vi "ResetAlarms.vi"(0 "reference in":refnum<class "Stand.lvclass">, 11 "error in (no error)":errorcluster) -> (4 "reference out":refnum<class "Stand.lvclass">, 15 "error out":errorcluster)   [LabVIEW 2019, in "Stand.lvclass"]
uses:
  Stand.lvclass
  Stand.lvclass/Stand.ctl
  Sig_AI_class/Sig_AI.lvclass
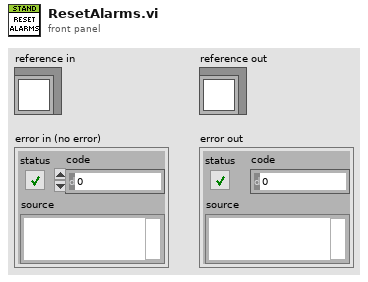
[diagram p1: front panel]
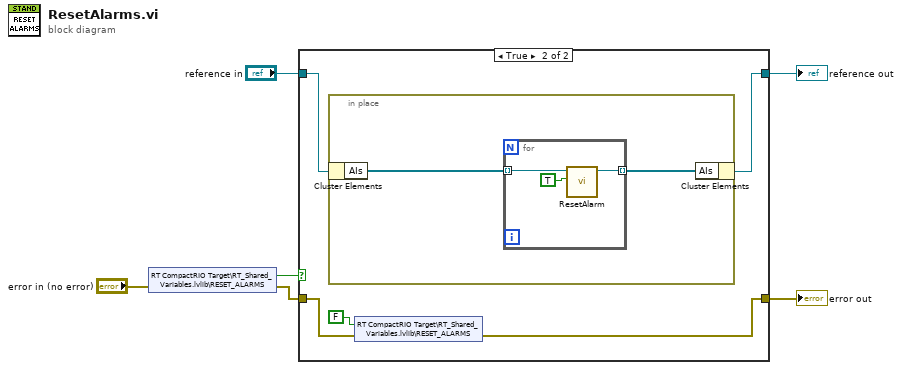
[diagram p0: block diagram]
diagram:
  n1 = shared-variable "RT CompactRIO Target\\RT_Shared_Variables.lvlib\\RESET_ALARMS"(error in="error in (no error)") -> (w2:bool, error out=w3:errorcluster)
  n2 = case shown="True" w2 {
    tunnel: w3 -> [w7 w12]
    tunnel: [w7 w11] -> w4
    tunnel: [w8 w9] -> w5
    tunnel: "reference in" -> [w8 w10]
    frame False {
    }
    frame True {
      n3 = in-place {
        n4 = in-place-cluster #1(w10) -> ("AIs"=w15:refnum<class "Sig_AI.lvclass">[])
        n5 = for {
          tunnel: w15 -> [w18] mode=indexing
          tunnel: [w17] -> w14 mode=indexing
          n6 = call "ResetAlarm.vi"("reset"=TRUE, "Sig_AI in"=w18) -> ("Sig_AI out"=w17:refnum<class "Sig_AI.lvclass">)  [unwired: 9 in]
        }
        n7 = in-place-cluster #1("AIs"=w14) -> (w9:refnum<class "Stand.lvclass">)
      }
      n8 = shared-variable "RT CompactRIO Target\\RT_Shared_Variables.lvlib\\RESET_ALARMS"(FALSE ("RESET_ALARMS"), error in=w12) -> (error out=w11:errorcluster)
    }
  }
  "reference out" <- w5
  "error out" <- w4
